vi "Downsampler_test.vi"(1 "No of points to average":i32, 2 "Input Array":dbl[](array[numeric]) format="%.2f") -> (0 "Downsampled Array":dbl[](array[numeric]) format="%.2f")   [LabVIEW 2011]
uses:
  <vilib>/Analysis/NI_AALBase.lvlib
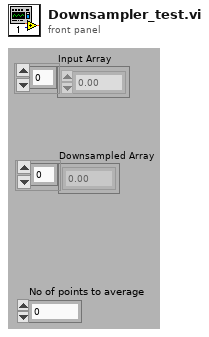
[diagram p1: front panel]
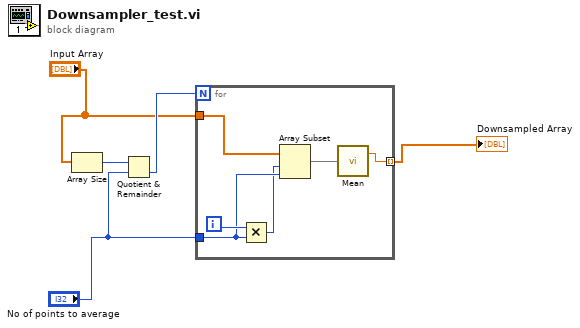
[diagram p0: block diagram]
diagram:
  n1 = Array Size(array="Input Array") -> (size(s)=w4:i32)
  n2 = Quotient & Remainder(x=w4, y="No of points to average") -> (floor(x/y)=w3:i32)  [unwired: 1 out]
  n3 = for {
    N: w3 -> [_]
    tunnel: "Input Array" -> [w11]
    tunnel: "No of points to average" -> [w9]
    tunnel: [w6] -> w1 mode=indexing
    i -> [w10]
    n4 = Multiply(x=w10, y=w9) -> (x*y=w8:i32)
    n5 = Array Subset(array=w11, index=w8, length=w9) -> (w7:dbl[])
    n6 = call <vilib>:"Mean.vi"("X"=w7) -> ("mean"=w6:dbl)  [unwired: 1 out]
  }
  "Downsampled Array" <- w1
